vi "DAQBasic.vi"() -> ()   [LabVIEW 2018]
uses:
  <vilib>/DAQmx/read.llb/DAQmx Read (Analog DBL 1Chan 1Samp).vi
  <vilib>/DAQmx/miscellaneous.llb/DAQmx Fill In Error Info.vi
panel:
  in  "stop":bool
  out "Waveform Chart":dbl(graph)
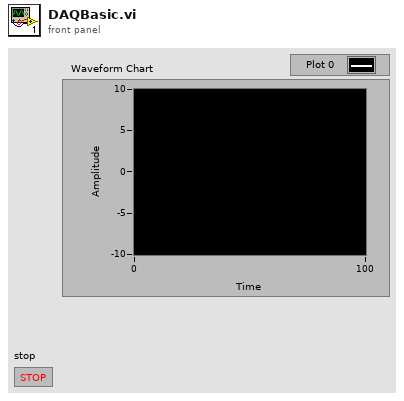
[diagram p1: front panel]
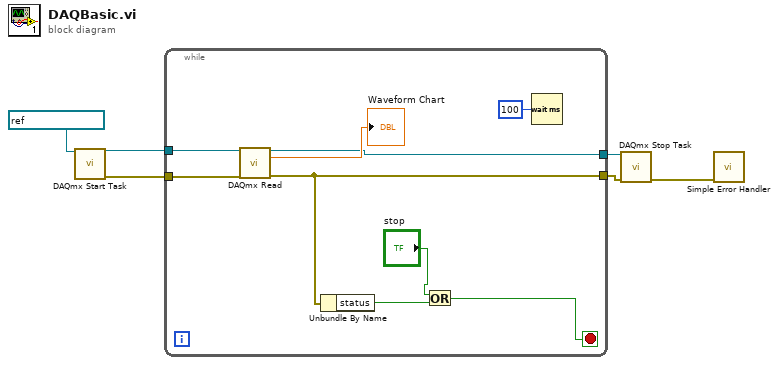
[diagram p0: block diagram]
diagram:
  n1 = call <vilib>:"DAQmx Start Task.vi"("task/channels in"=refnum<k21> "ADC-sisend0") -> ("task out"=w3:refnum<k21>, "error out"=w5:errorcluster)  [unwired: 13 in]
  n2 = while {
    tunnel: w5 -> [w14]
    tunnel: [w11] -> w4
    tunnel: w3 -> [w12]
    tunnel: [w7] -> w2
    stop <- w8 stop-if-true
    n3 = call-poly <vilib>:"DAQmx Read.vi"("task/channels in"=w12, "error in"=w14) -> ("task out"=w7:refnum<k21>, "data"=→"Waveform Chart":dbl, "error out"=w11:errorcluster)  [unwired: 11 in]
    n4 = Unbundle By Name(w11) -> ("status"=w10:bool)
    n5 = Or(x="stop", y=w10) -> (x .or. y?=w8:bool)
    n6 = Wait (ms)(milliseconds to wait=u32 100) -> ()  [unwired: 1 out]
  }
  n7 = call <vilib>:"DAQmx Stop Task.vi"("task/channels in"=w2, "error in"=w4) -> ("error out"=w1:errorcluster)  [unwired: 12 in, 1 out]
  n8 = call <vilib>:"Simple Error Handler.vi"("error in (no error)"=w1) -> ()  [unwired: 4 in, 5 out]
